vi "添加奶茶目录.vi"(8 "error in (no error)":errorcluster caption="错误输入（无错误）", 10 "奶茶.lvclass":refnum<class "奶茶.lvclass">, 11 "奶茶 输入":refnum<class "奶茶.lvclass">) -> (0 "error out":errorcluster caption="错误输出", 2 "奶茶目录名称":string[](array[string]), 3 "奶茶 输出":refnum<class "奶茶.lvclass">)   [LabVIEW 2016, in "奶茶.lvclass"]
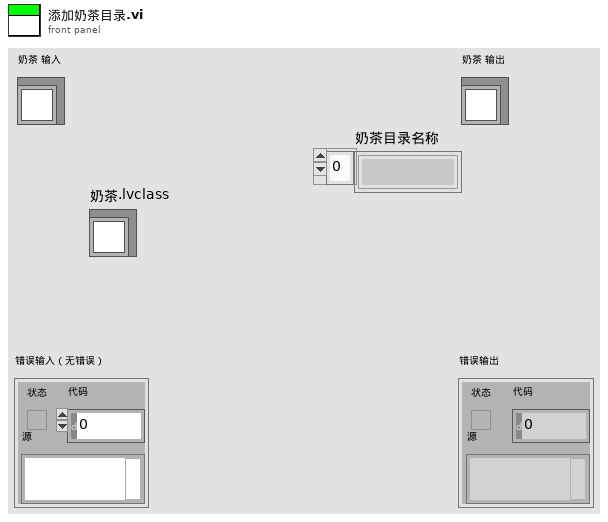
[diagram p1: front panel]
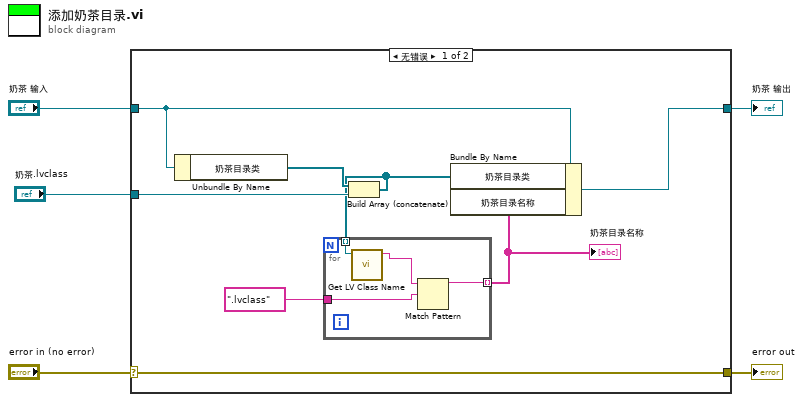
[diagram p0: block diagram]
diagram:
  n1 = case shown="无错误" "error in (no error)" {
    selector: "error in (no error)" -> [w13 w19]
    tunnel: [w13 w19] -> w4
    tunnel: [w12 w18] -> w2
    tunnel: "奶茶 输入" -> [w11 w18]
    tunnel: "奶茶.lvclass" -> [w9 _]
    frame No Error {
      n2 = Unbundle By Name(w11) -> ("奶茶目录类"=w10:refnum<class>[])
      n3 = Build Array (concatenate)(w10, w9) -> (w8:refnum<class>[])
      n4 = for {
        tunnel: w8 -> [w17] mode=indexing
        tunnel: ".lvclass" ("pattern") -> [w15]
        tunnel: [w14] -> w6 mode=indexing
        n5 = call <vilib>:"Get LV Class Name.vi"("object"=w17) -> ("class name"=w16:string)  [unwired: 9 in, 1 out]
        n6 = Match Pattern(string=w16, regular expression=w15) -> (before substring=w14:string)  [unwired: 1 in, 3 out]
      }
      "奶茶目录名称" <- w6
      n7 = Bundle By Name(cluster=w11, "奶茶目录类"=w8, "奶茶目录名称"=w6) -> (w12:refnum<class "奶茶.lvclass">)
    }
    frame Error {
    }
  }
  "error out" <- w4
  "奶茶 输出" <- w2
